vi "SubVI Tester.vi"() -> ()   [LabVIEW 2017]
uses:
  Weather Warnings/Weather Data.ctl
panel:
  in  "Min Temperature":dbl
  in  "Max Temperature":dbl
  out "Weather Data Out.":T1={"Current Temperature"=0.0, "Max Temperature"=0.0, "Min Temperature"=0.0, "Warning Text"="No Warning", "Temperature Warning?"=FALSE, "Current Windapeed"=0.0, "Max Windspeed"=0.0, "Windspeed Warning?"=FALSE, "Windspeed Warning text"="", "Units (0: Celsius)"=1} {"Units (0: Celsius)" items=["Celsius", "Fahrenheit"]}
  in  "Stop Button":bool
  in  "Weather Data In.":T1={"Current Temperature"=0.0, "Max Temperature"=0.0, "Min Temperature"=0.0, "Warning Text"="No Warning", "Temperature Warning?"=FALSE, "Current Windapeed"=0.0, "Max Windspeed"=0.0, "Windspeed Warning?"=FALSE, "Windspeed Warning text"="", "Units (0: Celsius)"=1} {"Units (0: Celsius)" items=["Celsius", "Fahrenheit"]}
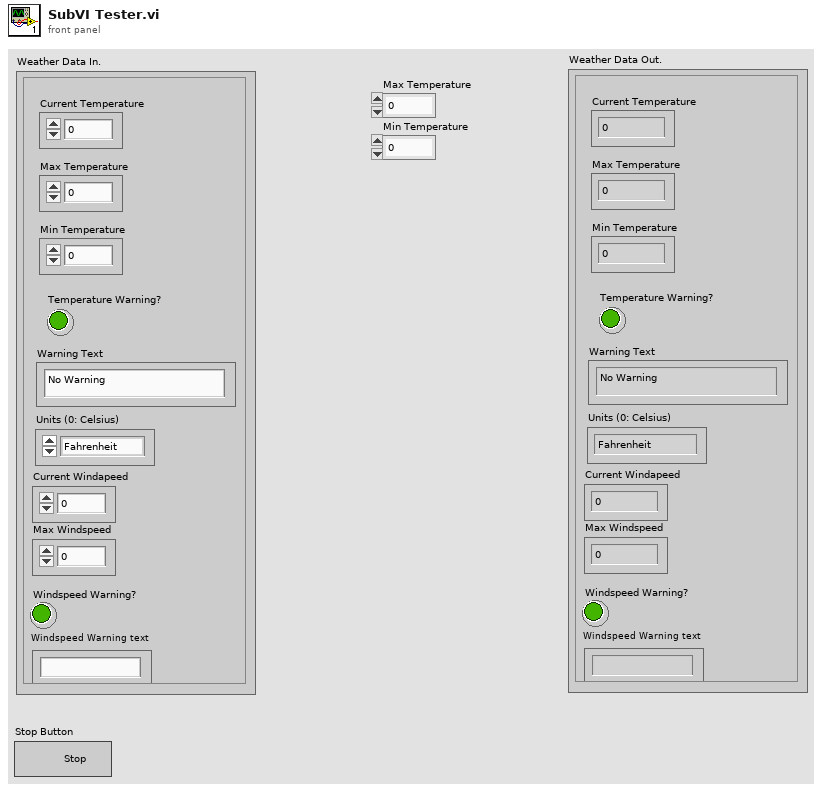
[diagram p1: front panel]
types:
  T1 = typedef "Weather Data.ctl" = cluster{"Current Temperature":dbl, "Max Temperature":dbl, "Min Temperature":dbl, "Warning Text":string, "Temperature Warning?":bool, "Current Windapeed":dbl, "Max Windspeed":dbl, "Windspeed Warning?":bool, "Windspeed Warning text":string, "Units (0: Celsius)":u16}
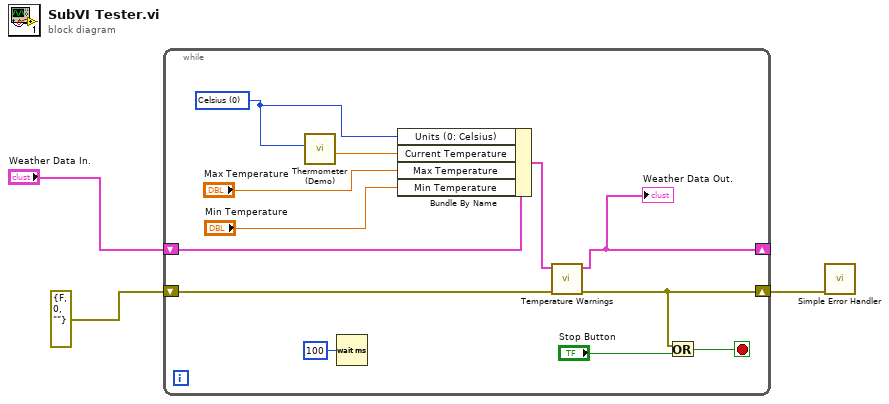
[diagram p0: block diagram]
diagram:
  n1 = while {
    shift-right: [w8] -> _
    shift-left: "Weather Data In." -> [w15]
    shift-right: [w11] -> w1
    shift-left: errorcluster {"status"=FALSE, "code"=0, "source"=""} ("error in (no error)") -> [w12]
    stop <- w9 stop-if-true
    w6 = u16 0 items=["Celsius", "Fahrenheit"] ("Units (0: Celsius)")
    n2 = call "Thermometer (Demo).vi"("Units (0: Celsius)"=w6) -> ("Temperature Value"=w14:dbl)  [unwired: 10 in]
    n3 = Wait (ms)(milliseconds to wait=u32 100) -> ()  [unwired: 1 out]
    n4 = Bundle By Name(cluster=w15, "Units (0: Celsius)"=w6, "Current Temperature"=w14, "Max Temperature"="Max Temperature", "Min Temperature"="Min Temperature") -> (w13:T1)
    n5 = call "Temperature Warnings.vi"("Error In"=w12, "Weather Data In."=w13) -> ("Error Out"=w11:errorcluster, "Weather Data Out."=w8:T1)  [unwired: 8 in]
    "Weather Data Out." <- w8
    n6 = Or(x=w11, y="Stop Button") -> (x .or. y?=w9:bool)
  }
  n7 = call <vilib>:"Simple Error Handler.vi"("error in (no error)"=w1) -> ()  [unwired: 4 in, 5 out]
